vi "Read userEvents.vi"(8 "error in (no error)":errorcluster, 11 "DataGridView in":refnum<class "DataGridView.lvclass">) -> (0 "error out":errorcluster, 2 "userEvents":T1, 3 "DataGridView out":refnum<class "DataGridView.lvclass">)   [LabVIEW 2013, in "DataGrid.lvlib" / "DataGridView.lvclass"]
uses:
  DataGridView.lvclass
  Events/Abstract EVENT/Abstract EVENT.lvclass
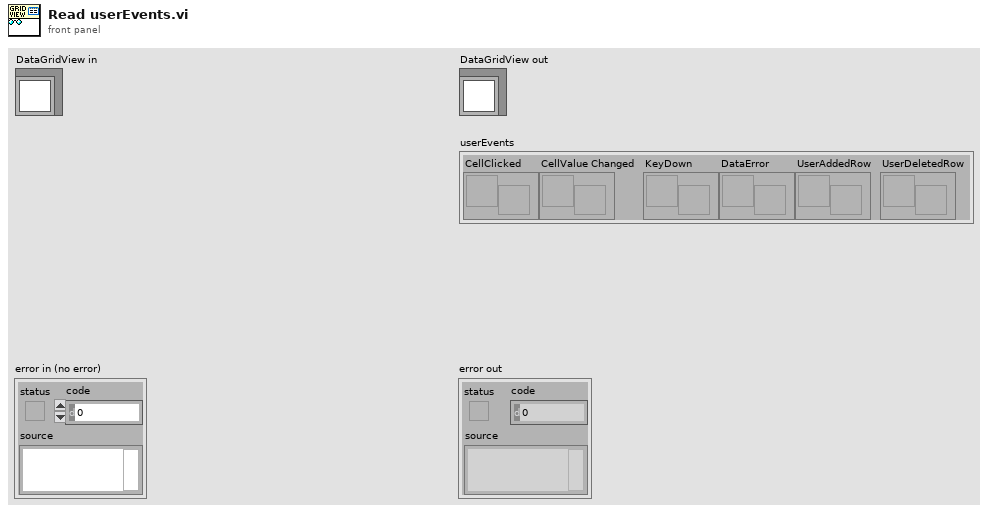
[diagram p1: front panel]
types:
  T1 = cluster{"CellClicked":refnum<user-event>, "CellValue Changed":refnum<user-event>, "KeyDown":refnum<user-event>, "DataError":refnum<user-event>, "UserAddedRow":refnum<user-event>, "UserDeletedRow":refnum<user-event>}
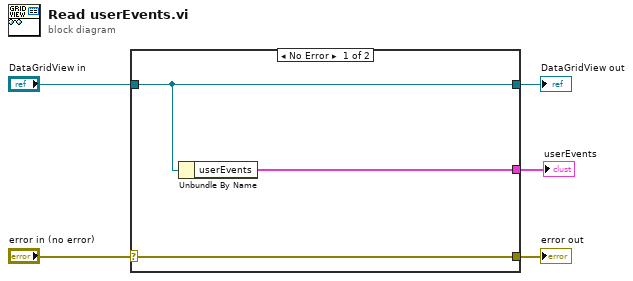
[diagram p0: block diagram]
diagram:
  n1 = case shown="No Error" "error in (no error)" {
    selector: "error in (no error)" -> [w8 w9]
    tunnel: [w8 w9] -> w4
    tunnel: [w7 w10] -> w2
    tunnel: "DataGridView in" -> [w7 w10]
    tunnel: [w6 _] -> w1
    frame No Error {
      n2 = Unbundle By Name(w7) -> ("userEvents"=w6:T1)
    }
    frame Error {
    }
  }
  "error out" <- w4
  "DataGridView out" <- w2
  "userEvents" <- w1
